vi "String To Hex(every bit).vi"(11 "字符串":string) -> (3 "十六进制整型字符串":string)   [LabVIEW 2017]
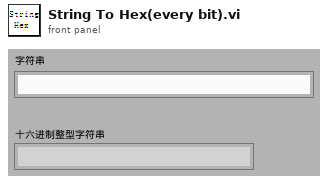
[diagram p1: front panel]
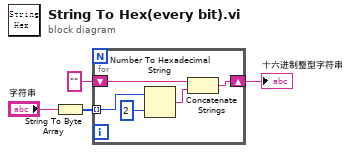
[diagram p0: block diagram]
diagram:
  n1 = String To Byte Array(string="字符串") -> (unsigned byte array=w3:u8[])
  n2 = for {
    tunnel: w3 -> [w9] mode=indexing
    shift-right: [w8] -> w2
    shift-left: "" -> [w7]
    n3 = Number To Hexadecimal String(1:i16 2 ("宽度(-)"), 2:w9) -> (0:w5:string)
    n4 = Concatenate Strings(w7, w5) -> (w8:string)
  }
  "十六进制整型字符串" <- w2
